vi "HelloWorld.vi"() -> ()   [LabVIEW 2019]
panel:
  out "String":string
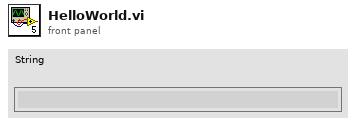
[diagram p1: front panel]
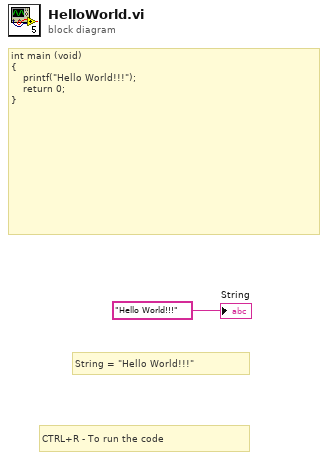
[diagram p0: block diagram]
diagram:
  # "CTRL+R - To run the code"
  # "String = \"Hello World!!!\""
  # "int main (void)\n{\n    printf(\"Hello World!!!\");\n    return 0;\n}"
  "String" <- "Hello World!!!"
